vi "svfa_Compute Zoom FFT (N Ch).vi"(0 "scaled signals [EU]":waveform(dbl)[](array[waveform]), 1 "processing control":T9(ring), 2 "spectra info in":T1[](array[typedef]) {"x-axis units" items=["Time (s)"=0, "Frequency-CB (Hz)"=1, "Frequency-CPB (Hz)"=1248, "Frequency-Arbitrary (Hz)"=2357, "Quefrency (s)"=2, "Revolutions (rev)"=3, "Order"=4, "Speed (RPM)"=11, "Speed (rad/s)"=21, "Index"=65535]; "weighting filter" items=["Linear", "A-weighting", "B-weighting", "C-weighting", "ITU-R 468-4", "Dolby", "CCITT", "C-message", "Wb", "Wc", "Wd", "We", "Wf", "Wh", "Wj", "Wk", "Wm", "AES17 20 kHz lowpass", "AES17 40 kHz lowpass", "AES17 20 kHz highpass", "AES17 40 kHz highpass"]; "dB reference [EU]" format="%.2f"; "engineering units" items=["custom..."=0, "V"=1, "A"=21, "C"=30, "pC"=31, "s"=32, "-"=29, "Pa"=2, "N"=20, "g"=3, "m/s^2"=4, "m/s"=5, "m"=6, "mm/s"=12, "mm"=13, "micron/s"=14, "micron"=15, "in/s^2"=7, "in/s"=8, "in"=9, "mil/s"=10, "mil"=11, "rad/s^2"=16, "rad/s"=17, "rad"=18, "deg/s^2"=26, "deg/s"=27, "deg"=28, "RPM"=22, "cycle/s^2"=23, "Hz"=24, "cycle"=25, "strain"=19]; "spectral info"."window" items=["None "=0, "Hanning"=1, "Hamming"=2, "Blackman-Harris"=3, "Exact Blackman"=4, "Blackman"=5, "Flat Top"=6, "4 Term B-Harris "=7, "7 Term B-Harris"=8, "Low Sidelobe"=9, "Force - Exponential"=10, "Gaussian"=62]}, 7 "maximum block size":i32, 9 "zoom FFT settings":T8={"zoom settings"={"center frequency"=-inf, "zoom"=1, "trim"=1.0}, "FFT settings"={"window"=enum."Hanning", "window size"=-1, "FFT size"=1024, "%overlap"=0.0}} {"FFT settings"."%overlap" min=0.0 max=100.0 format="%.2f"; "zoom settings"."trim" min=1.0 format="%.2f"; "zoom settings"."center frequency" format="%.2f"; "zoom settings"."zoom" min=1}, 11 "error in (no error)":errorcluster, 12 "iteration":i32, 13 "export time data?":bool) -> (3 "spectra info out":T1[](array[typedef]) {"x-axis units" items=["Time (s)"=0, "Frequency-CB (Hz)"=1, "Frequency-CPB (Hz)"=1248, "Frequency-Arbitrary (Hz)"=2357, "Quefrency (s)"=2, "Revolutions (rev)"=3, "Order"=4, "Speed (RPM)"=11, "Speed (rad/s)"=21, "Index"=65535]; "weighting filter" items=["Linear", "A-weighting", "B-weighting", "C-weighting", "ITU-R 468-4", "Dolby", "CCITT", "C-message", "Wb", "Wc", "Wd", "We", "Wf", "Wh", "Wj", "Wk", "Wm", "AES17 20 kHz lowpass", "AES17 40 kHz lowpass", "AES17 20 kHz highpass", "AES17 40 kHz highpass"]; "dB reference [EU]" format="%.2f"; "engineering units" items=["custom..."=0, "V"=1, "A"=21, "C"=30, "pC"=31, "s"=32, "-"=29, "Pa"=2, "N"=20, "g"=3, "m/s^2"=4, "m/s"=5, "m"=6, "mm/s"=12, "mm"=13, "micron/s"=14, "micron"=15, "in/s^2"=7, "in/s"=8, "in"=9, "mil/s"=10, "mil"=11, "rad/s^2"=16, "rad/s"=17, "rad"=18, "deg/s^2"=26, "deg/s"=27, "deg"=28, "RPM"=22, "cycle/s^2"=23, "Hz"=24, "cycle"=25, "strain"=19]; "spectral info"."window" items=["None "=0, "Hanning"=1, "Hamming"=2, "Blackman-Harris"=3, "Exact Blackman"=4, "Blackman"=5, "Flat Top"=6, "4 Term B-Harris "=7, "7 Term B-Harris"=8, "Low Sidelobe"=9, "Force - Exponential"=10, "Gaussian"=62]}, 4 "FFT spectra":cluster{"f0":dbl, "df":dbl, "spectrum":cdb[]}[](array[cluster]) {"spectrum" format="%.6g"; "df" format="%.2f"; "f0" format="%.2f"}, 10 "spectrum ready":bool, 14 "time data":T7(array[cluster]) {"data" format="%.2f"; "dt" format="%.2f"; "t0" format="%.2f"}, 15 "error out":errorcluster)   [LabVIEW 2017]
uses:
  <vilib>/addons/_NISVFA/_Shared subVIs/Controls/svc_Spectrum Info.ctl
  <vilib>/addons/_NISVFA/_Shared subVIs/Controls/svc_X-Axis Units.ctl
  <vilib>/addons/_NISVFA/_Shared subVIs/Controls/svc_Spectrum Type.ctl
  <vilib>/addons/_NISVFA/_Shared subVIs/Controls/svc_Engineering Units Text Ring.ctl
  <vilib>/addons/_NISVFA/_Shared subVIs/Controls/svc_Weighting Filter Text Ring.ctl
  <vilib>/addons/_NISVFA/_Shared subVIs/Controls/svc_Complimentary Spectrum Units.ctl
  <vilib>/Analysis/NI_AALPro.lvlib
  <vilib>/measure/NI_MAPro.lvlib
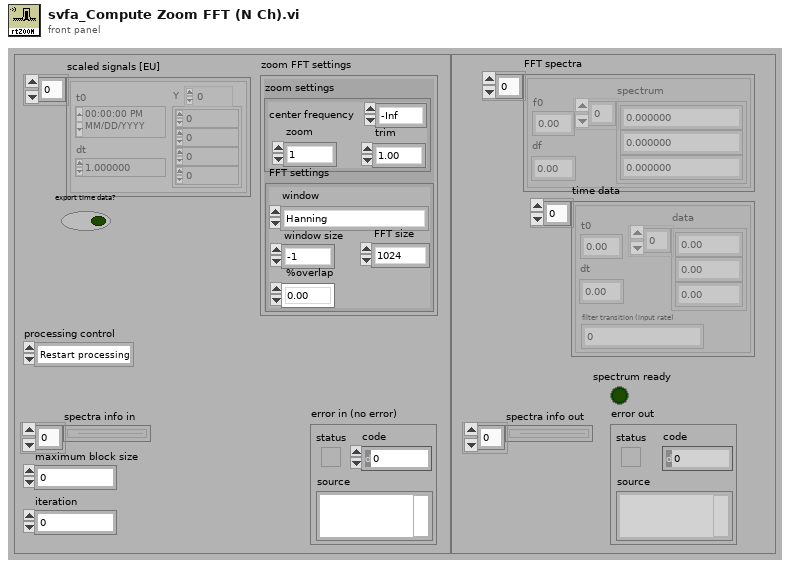
[diagram p1: front panel]
types:
  T1 = typedef "svc_Spectrum Info.ctl" = cluster{"channel name":string, "description":string, "x-axis units":T2, "spectral info":cluster{"spectrum type":T3, "linear/dB":enum16{"linear", "dB"}, "window":u16, "window size":i32, "FFT size":i32}, "engineering units":T4, "custom label":string, "dB reference [EU]":dbl, "peak units":enum16{"rms", "peak", "peak-peak"}, "weighting filter":T5, "spectral density?":bool, "unit label":string, "spectrum skewed?":bool, "complimentary spectrum units":T6}
  T2 = typedef "svc_X-Axis Units.ctl" = u16
  T3 = typedef "svc_Spectrum Type.ctl" = enum16{"FFT Spectrum [complex]", "Amplitude [Magnitude]", "Power [Magnitude^2]", "Cross Spectrum [complex]", "Frequency Response [Complex]"}
  T4 = typedef "svc_Engineering Units Text Ring.ctl" = u16
  T5 = typedef "svc_Weighting Filter Text Ring.ctl" = u16
  T6 = typedef "svc_Complimentary Spectrum Units.ctl" = enum16{"none", "radians", "degrees", "cycles", "imaginary"}
  T7 = cluster{"t0":dbl, "dt":dbl, "data":cdb[], "filter transition (input rate)":i32}[]
  T8 = cluster{"zoom settings":cluster{"center frequency":dbl, "zoom":i32, "trim":dbl}, "FFT settings":cluster{"window":enum16{"None ", "Hanning", "Hamming", "Blackman-Harris", "Exact Blackman", "Blackman", "Flat Top", "4 Term B-Harris ", "7 Term B-Harris", "Low Sidelobe"}, "window size":i32, "FFT size":i32, "%overlap":dbl}}
  T9 = enum16{"Restart processing", "Continue processing", "Skip processing"}
  T10 = cluster{"zoom":i32, "stop band attenuation":enum16{"84 dB", "96 dB", "120 dB"}, "alias protect in final transition":bool, "oversampling ratio":dbl}
  T11 = cluster{"t0":dbl, "dt":dbl, "data":cdb[], "filter transition (input rate)":i32}
  T12 = cluster{"window":enum16{"None ", "Hanning", "Hamming", "Blackman-Harris", "Exact Blackman", "Blackman", "Flat Top", "4 Term B-Harris ", "7 Term B-Harris", "Low Sidelobe"}, "window size":i32, "FFT size":i32, "%overlap":dbl}
  T13 = cluster{"zoom settings state":cluster{"zoom":i32, "stop band attenuation":enum16{"84 dB", "96 dB", "120 dB"}, "alias protect in final transition":bool, "oversampling ratio":dbl}, "SML Decimation Filter (complex input) state":cluster{"decimation settings state":cluster{"M":i32, "stop band attenuation":enum16{"84 dB", "96 dB", "120 dB"}, "alias protect in transition band":bool, "oversampling ratio":dbl}, "counter for garbage samples state":i32, "sml_Parameter Setting for Zoom Factor state":cluster{"filter length * interpolation state":i32, "interpolation state":i32, "comb filter order state":i32, "CFIR par state":cluster{"h":dbl[], "M":i32, "N":i32}, "LFIR par state":cluster{"h":dbl[], "M":i32, "N":i32}, "CIC Stages state":i32}, "aal_CIC (complex input) state":cluster{"aal_cascaded moving average (complex input) state":cluster{"states":cdb[], "circular buffers state":cdb[][], "circular buffer counter state":i32}, "aal_moving average with decimation by order (complex input) state":cluster{"residue result state":cdb, "processed data counter state":i32}}, "sml_Cascaded Decimation Filter (complex input) CFIR state":cluster{"unprocessed data state":cdb[], "final conditions state":cdb[][], "sml_M-1 Decimator with IC (complex input) state":cluster{"coefficients in reverse order state":dbl[], "max index for coefficients state":i32}}, "sml_Cascaded Decimation Filter (complex input) LFIR state":cluster{"unprocessed data state":cdb[], "final conditions state":cdb[][], "sml_M-1 Decimator with IC (complex input) state":cluster{"coefficients in reverse order state":dbl[], "max index for coefficients state":i32}}}, "ma_SML Data Packing (complex input) state":cluster{"array getting packed state":cdb[], "last array processed state":cdb[], "index state":i32, "packing parameters state":cluster{i32, "size":i32}}}
  T14 = cluster{"zoom settings state":cluster{"zoom":i32, "stop band attenuation":enum16{"84 dB", "96 dB", "120 dB"}, "alias protect in final transition":bool, "oversampling ratio":dbl}, "SML Decimation Filter (complex input) state":cluster{"decimation settings state":cluster{"M":i32, "stop band attenuation":enum16{"84 dB", "96 dB", "120 dB"}, "alias protect in transition band":bool, "oversampling ratio":dbl}, "counter for garbage samples state":i32, "sml_Parameter Setting for Zoom Factor state":cluster{"filter length * interpolation state":i32, "interpolation state":i32, "comb filter order state":i32, "CFIR par state":cluster{"h":dbl[], "M":i32, "N":i32}, "LFIR par state":cluster{"h":dbl[], "M":i32, "N":i32}, "CIC Stages state":i32}, "aal_CIC (complex input) state":cluster{"aal_cascaded moving average (complex input) state":cluster{"states":cdb[], "circular buffers state":cdb[][], "circular buffer counter state":i32}, "aal_moving average with decimation by order (complex input) state":cluster{"residue result state":cdb, "processed data counter state":i32}}, "sml_Cascaded Decimation Filter (complex input) CFIR state":cluster{"unprocessed data state":cdb[], "final conditions state":cdb[][], "sml_M-1 Decimator with IC (complex input) state":cluster{"coefficients in reverse order state":dbl[], "max index for coefficients state":i32}}, "sml_Cascaded Decimation Filter (complex input) LFIR state":cluster{"unprocessed data state":cdb[], "final conditions state":cdb[][], "sml_M-1 Decimator with IC (complex input) state":cluster{"coefficients in reverse order state":dbl[], "max index for coefficients state":i32}}}, "ma_SML Data Packing (complex input) state":cluster{"array getting packed state":cdb[], "last array processed state":cdb[], "index state":i32, "packing parameters state":cluster{i32, "size":i32}}}[]
  T15 = typedef "NI_MAPro.lvlib/ma_sml_Spectral Info.ctl" = cluster{"spectrum type":enum16{"FFT Spectrum [complex]", "Amplitude [Magnitude]", "Power [Magnitude^2]", "Cross Spectrum [complex]", "Frequency Response [Complex]"}, "linear/dB":enum16{"linear", "dB"}, "window":u16, "window size":i32, "FFT size":i32}
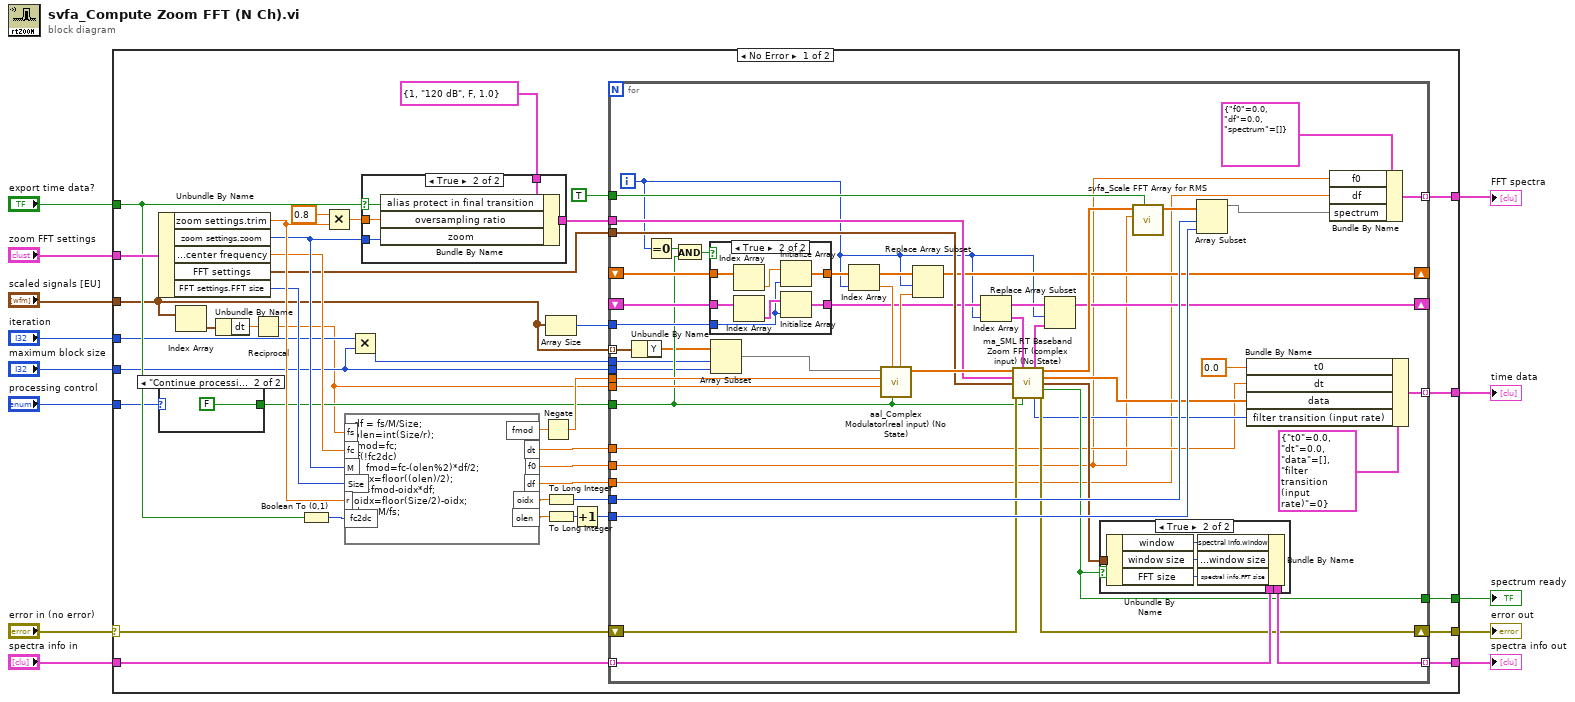
[diagram p0: block diagram]
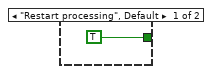
[diagram p4: hidden frame]
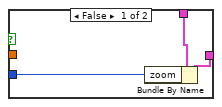
[diagram p5: hidden frame]
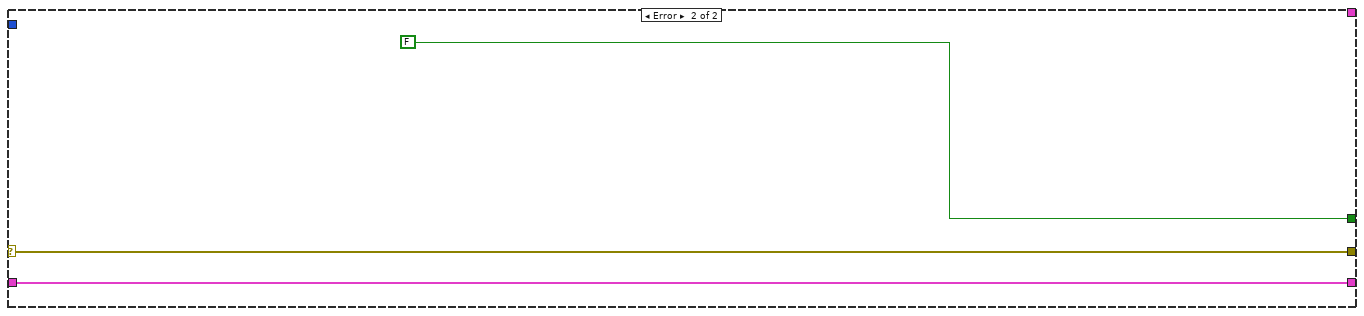
[diagram p6: hidden frame]
diagram:
  n1 = case shown="No Error" "error in (no error)" {
    selector: "error in (no error)" -> [w25 w128]
    tunnel: [w52 _] -> w9
    tunnel: [w23 FALSE ("SpectrumReady")] -> w13
    tunnel: "scaled signals [EU]" -> [w17 _]
    tunnel: [w53 _] -> w12
    tunnel: "spectra info in" -> [w31 w127]
    tunnel: [w30 w127] -> w7
    tunnel: [w24 w128] -> w6
    tunnel: "zoom FFT settings" -> [w51 _]
    tunnel: "processing control" -> [w29 _]
    tunnel: "export time data?" -> [w50 _]
    tunnel: "maximum block size" -> [w19 _]
    tunnel: "iteration" -> [w20 _]
    frame No Error {
      n2 = Unbundle By Name(w51) -> ("zoom settings.trim"=w35:dbl, "zoom settings.zoom"=w33:i32, "zoom settings.center frequency"=w32:dbl, "FFT settings"=w22:T12, "FFT settings.FFT size"=w34:i32)
      n3 = case shown="\"Continue processing\", \"Skip processing\"" w29 {
        tunnel: [TRUE FALSE] -> w26
        frame "Restart processing", Default {
        }
        frame "Continue processing", "Skip processing" {
        }
      }
      n4 = Index Array(array=w17) -> (element=w16:waveform(dbl))  [unwired: 1 in]
      n5 = Unbundle By Name(w16) -> ("dt"=w15:dbl)
      n6 = Reciprocal(x=w15) -> (1/x=w14:dbl)
      n7 = Boolean To (0,1)(Boolean=w50) -> (0, 1=w36:i16)
      n8 = Multiply(x=0.8, y=w35) -> (x*y=w39:dbl)
      n9 = formula code="df = fs/M/Size;\nolen=int(Size/r);\nfmod=fc;\nif(!fc2dc)\n    fmod=fc-(olen%2)*df/2;\noidx=floor((olen)/2);\nf0=fmod-oidx*df;\noidx=floor(Size/2)-oidx;\ndt = M/fs;"("fc"=w32, "M"=w33, "Size"=w34, "fs"=w14, "r"=w35, "fc2dc"=w36) -> ("f0"=w27:dbl, "df"=w49:dbl, "oidx"=w48:dbl, "olen"=w47:dbl, "dt"=w41:dbl, "fmod"=w37:dbl)
      n10 = Multiply(x=w20, y=w19) -> (x*y=w18:i32)
      n11 = case shown="True" w50 {
        selector: w50 -> [_ w124]
        tunnel: T10 {"zoom"=1, "stop band attenuation"=enum."120 dB", "alias protect in final transition"=FALSE, "oversampling ratio"=1.0} ("zoom settings") -> [w121 w126]
        tunnel: [w120 w125] -> w42
        tunnel: w33 -> [w119 w122]
        tunnel: w39 -> [_ w123]
        frame False {
          n12 = Bundle By Name(cluster=w121, "zoom"=w119) -> (w120:T10)
        }
        frame True {
          n13 = Bundle By Name(cluster=w126, "alias protect in final transition"=w124, "oversampling ratio"=w123, "zoom"=w122) -> (w125:T10)
        }
      }
      n14 = Negate(x=w37) -> (-x=w44:dbl)
      n15 = Array Size(array=w17) -> (size(s)=w21:i32)
      n16 = To Long Integer(number=w48) -> (32bit integer=w46:i32)
      n17 = To Long Integer(number=w47) -> (32bit integer=w45:i32)
      n18 = Increment(x=w45) -> (x+1=w40:i32)
      n19 = for {
        tunnel: w17 -> [w100] mode=indexing
        tunnel: [w54] -> w53 mode=indexing
        tunnel: w14 -> [w99]
        tunnel: [w60] -> w52 mode=indexing
        tunnel: w49 -> [w56]
        tunnel: w46 -> [w96]
        tunnel: w44 -> [w95]
        tunnel: w42 -> [w94]
        tunnel: w41 -> [w61]
        tunnel: w40 -> [w93]
        tunnel: w22 -> [w91]
        tunnel: w31 -> [w90] mode=indexing
        tunnel: [w89] -> w30 mode=indexing
        tunnel: TRUE -> [w87]
        tunnel: w27 -> [w57]
        tunnel: w26 -> [w70]
        tunnel: [w84] -> w23
        shift-right: [w85] -> w24
        shift-left: w25 -> [w86]
        shift-right: [w81] -> _
        shift-left: _ -> [w77]
        shift-right: [w80] -> _
        shift-left: _ -> [w76]
        tunnel: w21 -> [w73]
        tunnel: w19 -> [w66]
        tunnel: w18 -> [w65]
        i -> [w71]
        n20 = Unbundle By Name(w100) -> ("Y"=w68:dbl[])
        n21 = Equal To 0?(x=w71) -> (x = 0?=w72:bool)
        n22 = And(x=w72, y=w70) -> (x .and. y?=w69:bool)
        n23 = case shown="True" w69 {
          tunnel: w77 -> [w102 w109]
          tunnel: w76 -> [w101 w108]
          tunnel: [w102 w106] -> w75
          tunnel: [w101 w105] -> w74
          tunnel: w73 -> [_ w103]
          frame False {
          }
          frame True {
            n24 = Index Array(array=w109) -> (element=w104:dbl)  [unwired: 1 in]
            n25 = Index Array(array=w108) -> (element=w107:T13)  [unwired: 1 in]
            n26 = Initialize Array(w104, w103) -> (w106:dbl[])
            n27 = Initialize Array(w107, w103) -> (w105:T14)
          }
        }
        n28 = Array Subset(array=w68, index=w65, length=w66) -> (w67:dbl[])
        n29 = Index Array(array=w75, index=w71) -> (element=w83:dbl)
        n30 = call <vilib>:"aal_Complex Modulator(real input) (No State).vi"("reset ?"=w70, "initial phase"=w83, "fs"=w99, "frequency"=w95, "x"=w67) -> ("y"=w97:cdb[], "next initial phase"=w82:dbl)  [unwired: 5 in]
        n31 = Replace Array Subset(array=w75, new element=w82, index=w71) -> (w81:dbl[])
        n32 = Index Array(array=w74, index=w71) -> (element=w79:T13)
        n33 = call <vilib>:"ma_SML RT Baseband Zoom FFT (complex input) (No State).vi"("x [V]"=w97, "SML RT Baseband Zoom FFT (complex input) state in"=w79, "zoom settings"=w94, "FFT settings"=w91, "error in (no error)"=w86, "reset?"=w70) -> ("SML RT Baseband Zoom FFT (complex input) state out"=w78:T13, "FFT{X} [Vrms]"=w98:cdb[], "time data"=w64:cdb[], "spectral info"=w88:T15, "spectrum ready?"=w84:bool, "filter transition length"=w63:i32, "error out"=w85:errorcluster)  [unwired: 3 in]
        n34 = Replace Array Subset(array=w74, new element=w78, index=w71) -> (w80:T14)
        n35 = case shown="True" w84 {
          tunnel: w90 -> [w110 w116]
          tunnel: [w110 w115] -> w89
          tunnel: w88 -> [_ w114]
          frame False {
          }
          frame True {
            n36 = Unbundle By Name(w114) -> ("window"=w113:u16, "window size"=w112:i32, "FFT size"=w111:i32)
            n37 = Bundle By Name(cluster=w116, "spectral info.window"=w113, "spectral info.window size"=w112, "spectral info.FFT size"=w111) -> (w115:T1)
          }
        }
        n38 = call <vilib>:"svfa_Scale FFT Array for RMS.vi"("leave DC bin unscaled (T)"=w87, "f0"=w57, "FFT{X} [EU]"=w98) -> ("FFT {X} [rms]"=w92:cdb[])  [unwired: 8 in]
        n39 = Array Subset(array=w92, index=w96, length=w93) -> (w55:cdb[])
        n40 = Bundle By Name(cluster=T11 {"t0"=0.0, "dt"=0.0, "data"=[], "filter transition (input rate)"=0} ("time data"), "t0"=0.0 ("x"), "dt"=w61, "data"=w64, "filter transition (input rate)"=w63) -> (w60:T11)
        n41 = Bundle By Name(cluster=cluster{"f0":dbl, "df":dbl, "spectrum":cdb[]} {"f0"=0.0, "df"=0.0, "spectrum"=[]} ("FFT spectrum"), "f0"=w57, "df"=w56, "spectrum"=w55) -> (w54:cluster{"f0":dbl, "df":dbl, "spectrum":cdb[]})
      }
    }
    frame Error {
    }
  }
  "spectrum ready" <- w13
  "FFT spectra" <- w12
  "error out" <- w6
  "time data" <- w9
  "spectra info out" <- w7
